vi "Get Property Type.vi"(8 "error in":errorcluster, 11 "Node in":refnum<k20>) -> (0 "error out":errorcluster, 2 "Type":T1(ring)=enum."DictionaryArray", 3 "Node out":refnum<k20>, 4 "Enum TypeName":string)   [LabVIEW 2026, in "Plugin XML Parser.lvlib"]
uses:
  Plugin XML Parser.lvlib
  <resource>/objmgr/DOMUserDefRef.rc
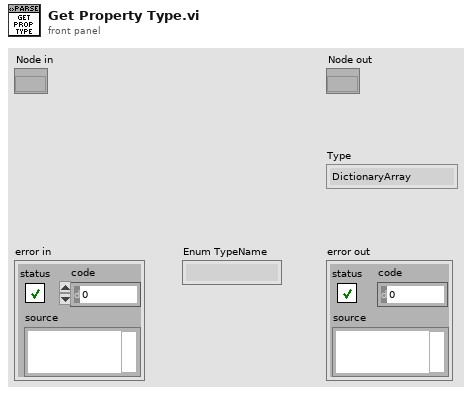
[diagram p1: front panel]
types:
  T1 = enum16{"String", "BinaryString", "Boolean", "I32", "I16", "I64", "U32", "U16", "Double", "U64", "Variant", "DependentNode", "DataSourceNode", "DependentFile", "BooleanArray", "U64Array", "U32Array", "U16Array", "DoubleArray", "I64Array", "I32Array", "I16Array", "StringArray", "Enum", "Dictionary", "DictionaryArray", "None"}
  T2 = enum16{"String", "BinaryString", "Boolean", "I32", "I16", "I64", "U32", "U16", "Double", "U64", "Variant", "DependentNode", "DataSourceNode", "DependentFile", "BooleanArray", "U64Array", "U32Array", "U16Array", "DoubleArray", "I64Array", "I32Array", "I16Array", "StringArray", "Dictionary", "DictionaryArray", "None"}
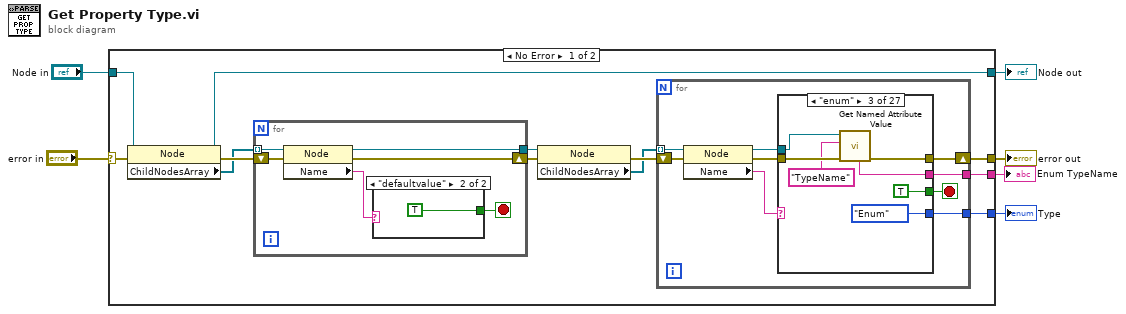
[diagram p0: block diagram]
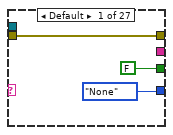
[diagram p2: hidden frame]
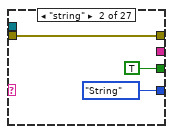
[diagram p3: hidden frame]
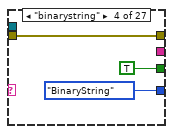
[diagram p4: hidden frame]
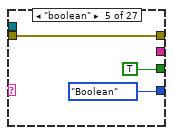
[diagram p5: hidden frame]
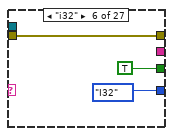
[diagram p6: hidden frame]
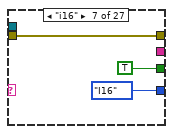
[diagram p7: hidden frame]
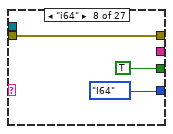
[diagram p8: hidden frame]
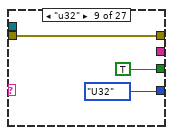
[diagram p9: hidden frame]
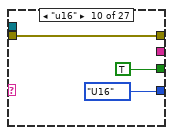
[diagram p10: hidden frame]
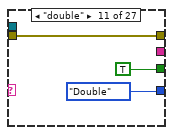
[diagram p11: hidden frame]
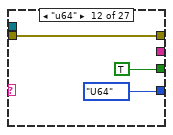
[diagram p12: hidden frame]
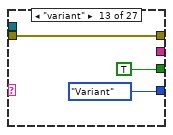
[diagram p13: hidden frame]
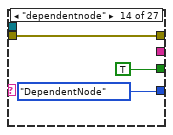
[diagram p14: hidden frame]
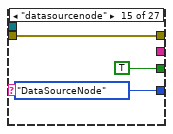
[diagram p15: hidden frame]
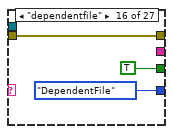
[diagram p16: hidden frame]
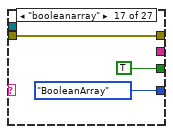
[diagram p17: hidden frame]
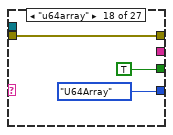
[diagram p18: hidden frame]
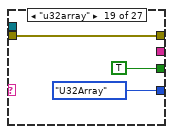
[diagram p19: hidden frame]
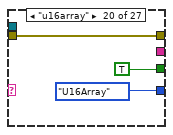
[diagram p20: hidden frame]
diagram:
  n1 = case shown="No Error" "error in" {
    selector: "error in" -> [w18 w122]
    tunnel: [w14 w122] -> w6
    tunnel: [w12 w121] -> w4
    tunnel: "Node in" -> [w13 w121]
    tunnel: [w8 _] -> w2
    tunnel: [w7 _] -> w1
    frame No Error {
      n2 = property class="Node"(reference=w13, error in=w18) -> (reference out=w12:refnum<k20>, error out=w17:errorcluster, "ChildNodesArray"=w11:refnum<k20>[])
      n3 = for {
        tunnel: w11 -> [w116] mode=indexing
        shift-right: [w117] -> w16
        shift-left: w17 -> [w118]
        tunnel: [w113] -> w10
        stop <- w114 stop-if-true
        n4 = property class="Node"(reference=w116, error in=w118) -> (reference out=w113:refnum<k20>, error out=w117:errorcluster, "Name"=w115:string)
        n5 = case shown="\"defaultvalue\"" w115 {
          tunnel: [FALSE TRUE] -> w114
          frame Default {
          }
          frame "defaultvalue" {
          }
        }
      }
      n6 = property class="Node"(reference=w10, error in=w16) -> (error out=w15:errorcluster, "ChildNodesArray"=w9:refnum<k20>[])  [unwired: 1 out]
      n7 = for {
        tunnel: w9 -> [w26] mode=indexing
        tunnel: [w24] -> w8
        shift-right: [w20] -> w14
        shift-left: w15 -> [w27]
        tunnel: [w19] -> w7
        stop <- w23 stop-if-true
        n8 = property class="Node"(reference=w26, error in=w27) -> (reference out=w21:refnum<k20>, error out=w22:errorcluster, "Name"=w25:string)
        n9 = case shown="\"enum\"" w25 {
          tunnel: [T2."None" T2."String" T1."Enum" T2."BinaryString" T2."Boolean" T2."I32" T2."I16" T2."I64" T2."U32" T2."U16" T2."Double" T2."U64" T2."Variant" T2."DependentNode" T2."DataSourceNode" T2."DependentFile" T2."BooleanArray" T2."U64Array" T2."U32Array" T2."U16Array" T2."DoubleArray" T2."I64Array" T2."I32Array" T2."I16Array" T2."StringArray" T2."Dictionary" T2."DictionaryArray"] -> w24
          tunnel: [FALSE TRUE TRUE TRUE TRUE TRUE TRUE TRUE TRUE TRUE TRUE TRUE TRUE TRUE TRUE TRUE TRUE TRUE TRUE TRUE TRUE TRUE TRUE TRUE TRUE TRUE TRUE] -> w23
          tunnel: w22 -> [w28 w31 w37 w41 w44 w47 w50 w53 w56 w59 w62 w65 w68 w71 w74 w77 w80 w83 w86 w89 w92 w95 w98 w101 w104 w107 w110]
          tunnel: w21 -> [_ _ w38 _ _ _ _ _ _ _ _ _ _ _ _ _ _ _ _ _ _ _ _ _ _ _ _]
          tunnel: [w28 w31 w35 w41 w44 w47 w50 w53 w56 w59 w62 w65 w68 w71 w74 w77 w80 w83 w86 w89 w92 w95 w98 w101 w104 w107 w110] -> w20
          tunnel: [_ _ w34 _ _ _ _ _ _ _ _ _ _ _ _ _ _ _ _ _ _ _ _ _ _ _ _] -> w19
          frame Default {
          }
          frame "string" {
          }
          frame "enum" {
            n10 = call "Get Named Attribute Value.vi"("error in"=w37, "Attribute Name"="TypeName", "Node In"=w38) -> ("error out"=w35:errorcluster, "Attribute Value"=w34:string)  [unwired: 5 in, 2 out]
          }
          frame "binarystring" {
          }
          frame "boolean" {
          }
          frame "i32" {
          }
          frame "i16" {
          }
          frame "i64" {
          }
          frame "u32" {
          }
          frame "u16" {
          }
          frame "double" {
          }
          frame "u64" {
          }
          frame "variant" {
          }
          frame "dependentnode" {
          }
          frame "datasourcenode" {
          }
          frame "dependentfile" {
          }
          frame "booleanarray" {
          }
          frame "u64array" {
          }
          frame "u32array" {
          }
          frame "u16array" {
          }
          frame "doublearray" {
          }
          frame "i64array" {
          }
          frame "i32array" {
          }
          frame "i16array" {
          }
          frame "stringarray" {
          }
          frame "dictionary" {
          }
          frame "dictionaryarray" {
          }
        }
      }
    }
    frame Error {
    }
  }
  "Node out" <- w4
  "error out" <- w6
  "Type" <- w2
  "Enum TypeName" <- w1
